vi "quiensabequehacerconesto.vi"() -> ()   [LabVIEW 2021]
uses:
  <vilib>/vision/Image Controls.llb/IMAQ Image.ctl
  <vilib>/vision/NI_Vision_Development_Module.lvlib
panel:
  out "Patrón corregido":T1(plugin-control) caption="Perfil lateral"
  in  "Toma original":T1
  in  "Patrón 3":T1
  out "Patrón 2":cluster{"X Centroid":sgl, "Y Centroid":sgl} {"Y Centroid" format="%.2f"; "X Centroid" format="%.2f"}
  out "Toma":cluster{"X Centroid":sgl, "Y Centroid":sgl} {"Y Centroid" format="%.2f"; "X Centroid" format="%.2f"}
  out "Centroide coregido":cluster{"X Centroid":sgl, "Y Centroid":sgl} {"Y Centroid" format="%.2f"; "X Centroid" format="%.2f"}
  out "Angulo corregido":dbl format="%.2f"
  out "Angulo no corregido":dbl format="%.2f"
  out "Toma Cámara":T1(plugin-control) caption="Perfil lateral"
  out "Patrón":T1(plugin-control) caption="Perfil lateral"
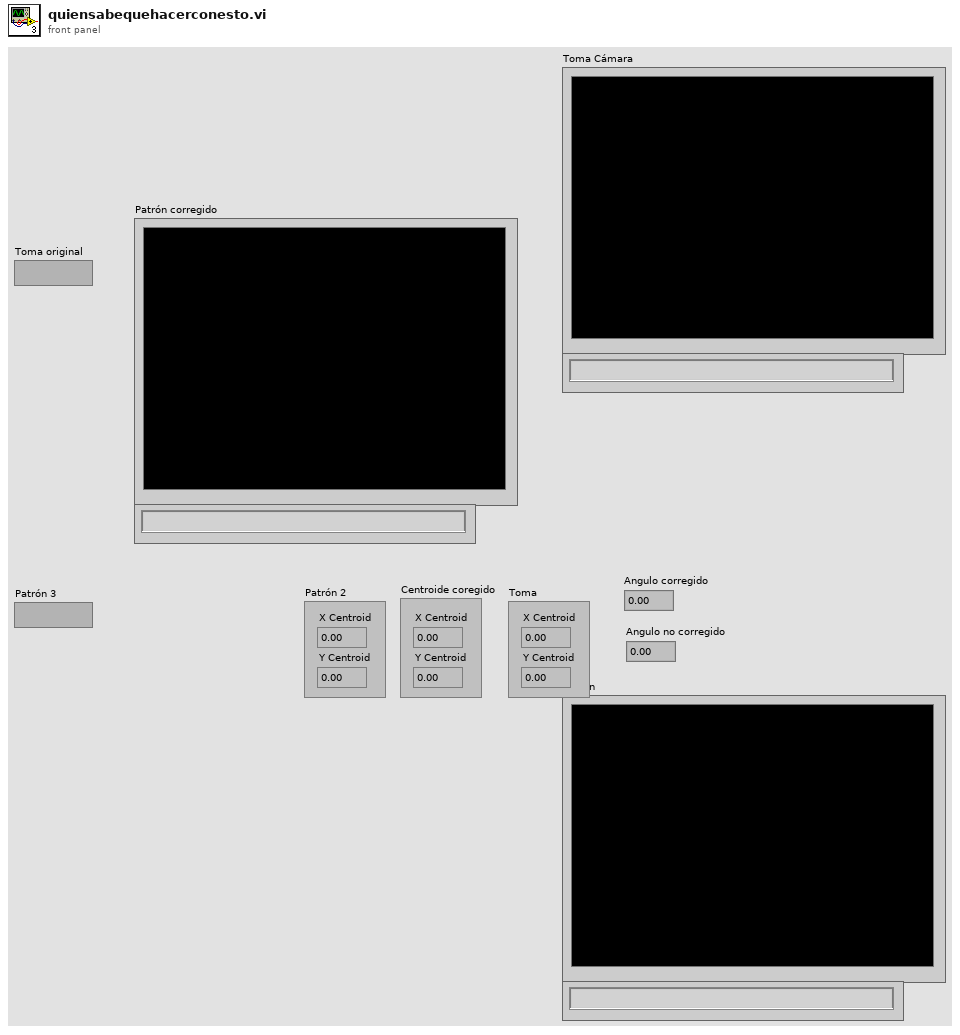
[diagram p1: front panel]
types:
  T1 = typedef "IMAQ Image.ctl" = refnum<image>
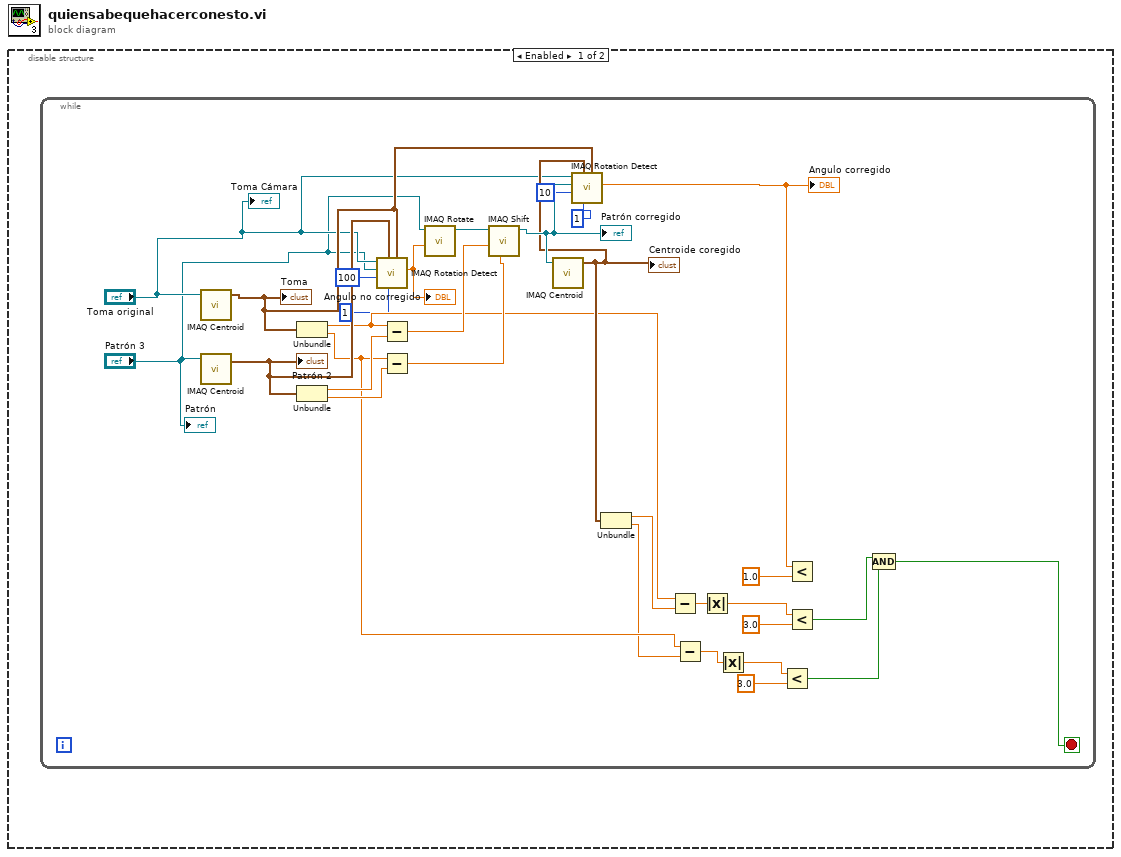
[diagram p0: block diagram]
diagram:
  n1 = disable-structure shown="Enabled" {
    frame Enabled {
      n2 = while {
        stop <- w30 stop-if-true
        n3 = call "IMAQ Centroid"("Image"="Toma original") -> ("Centroid"=w14:cluster{"X Centroid":sgl, "Y Centroid":sgl})  [unwired: 3 in, 1 out]
        "Toma" <- w14
        n4 = call "IMAQ Centroid"("Image"="Patrón 3") -> ("Centroid"=w20:cluster{"X Centroid":sgl, "Y Centroid":sgl})  [unwired: 3 in, 1 out]
        "Patrón 2" <- w20
        n5 = Unbundle(w14) -> ("X Centroid"=w11:sgl, "Y Centroid"=w10:sgl)
        n6 = Unbundle(w20) -> ("X Centroid"=w19:sgl, "Y Centroid"=w18:sgl)
        n7 = call "IMAQ Rotation Detect"("Reference Center"=w14, "Precision (degrees)"=1, "Image 2 Center"=w20, "Radius"=100, "Image 2"="Patrón 3", "Reference Image"="Toma original") -> ("Angle (deg)"=w1:dbl)  [unwired: 3 in, 2 out]
        "Angulo no corregido" <- w1
        n8 = Subtract(x=w11, y=w19) -> (x-y=w17:sgl)
        n9 = Subtract(x=w10, y=w18) -> (x-y=w16:sgl)
        n10 = call "IMAQ Rotate"("Angle (degrees)"=w1, "Image Src"="Patrón 3") -> ("Image Dst Out"=w31:T1)  [unwired: 8 in, 1 out]
        n11 = call "IMAQ Shift"("YOffset"=w16, "XOffset"=w17, "Image Src"=w31) -> ("Image Dst Out"=w15:T1)  [unwired: 7 in, 1 out]
        "Patrón corregido" <- w15
        n12 = call "IMAQ Centroid"("Image"=w15) -> ("Centroid"=w13:cluster{"X Centroid":sgl, "Y Centroid":sgl})  [unwired: 3 in, 1 out]
        "Centroide coregido" <- w13
        n13 = call "IMAQ Rotation Detect"("Reference Center"=w14, "Precision (degrees)"=1, "Image 2 Center"=w13, "Radius"=10, "Image 2"=w15, "Reference Image"="Toma original") -> ("Angle (deg)"=w12:dbl)  [unwired: 3 in, 2 out]
        "Angulo corregido" <- w12
        n14 = Unbundle(w13) -> ("X Centroid"=w9:sgl, "Y Centroid"=w8:sgl)
        n15 = Subtract(x=w11, y=w9) -> (x-y=w24:sgl)
        n16 = Subtract(x=w10, y=w8) -> (x-y=w23:sgl)
        n17 = Absolute Value(x=w24) -> (abs(x)=w21:sgl)
        n18 = Absolute Value(x=w23) -> (abs(x)=w22:sgl)
        n19 = Less?(x=w22, y=3.0) -> (x < y?=w25:bool)
        n20 = Less?(x=w12, y=1.0) -> ()  [unwired: 1 out]
        n21 = Less?(x=w21, y=3.0) -> (x < y?=w26:bool)
        n22 = Compound Arithmetic op=AND(w26, w25) -> (w30:bool)
        "Toma Cámara" <- "Toma original"
        "Patrón" <- "Patrón 3"
      }
    }
    frame Disabled {
    }
  }
